vi "写入差值数据excel.vi"(7 "IN":i32=129, 8 "error in (no error)":errorcluster, 9 "COM":i32=4, 10 "差值限":dbl, 11 "NI_report in":refnum<class "NI_report.lvclass">) -> (0 "error out":errorcluster, 3 "NI_report out":refnum<class "NI_report.lvclass">)   [LabVIEW 2015]
uses:
  <vilib>/Utility/NIReport.llb/NI_report.lvclass
  <vilib>/addons/_office/excel.llb/Excel Easy Table (str).vi
  <vilib>/Utility/NIReport.llb/Excel/NI_Excel.lvclass
  <vilib>/addons/_office/NI_ReportGenerationToolkit.lvlib
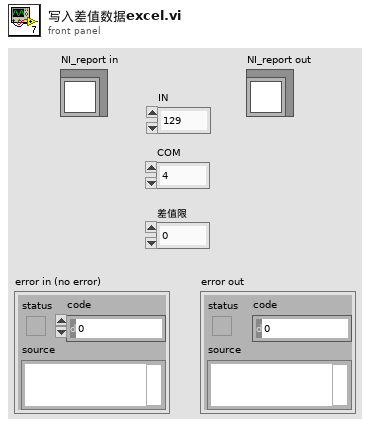
[diagram p1: front panel]
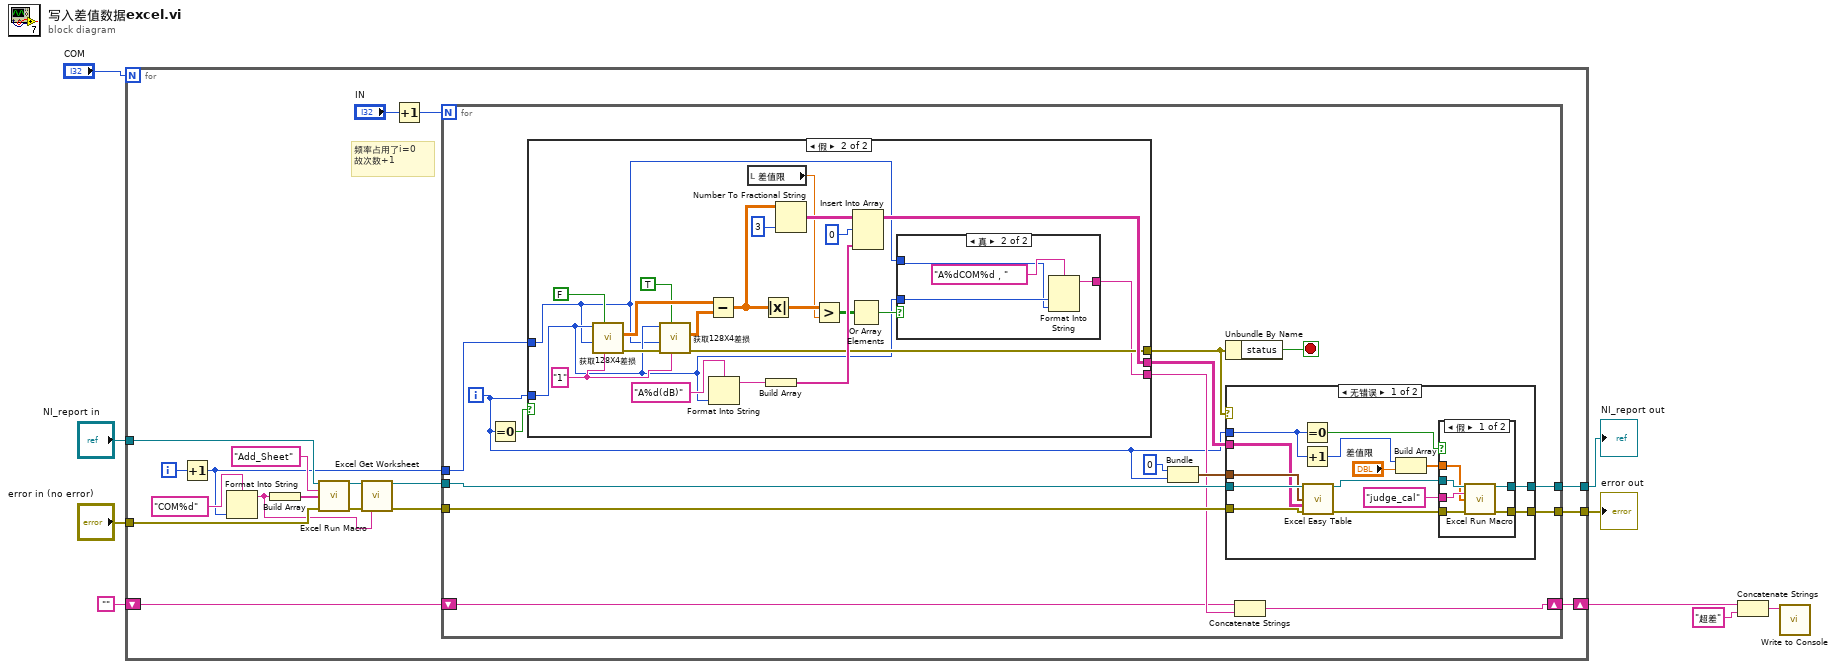
[diagram p0: block diagram]
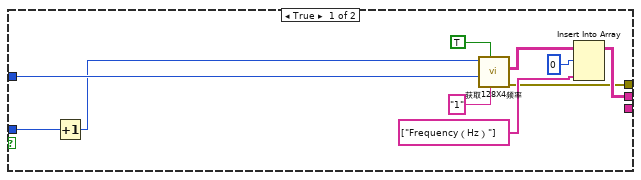
[diagram p2: hidden frame]
diagram:
  n1 = for {
    N: "COM" -> [_]
    tunnel: "NI_report in" -> [w25]
    tunnel: "error in (no error)" -> [w24]
    tunnel: [w14] -> w8
    tunnel: [w13] -> w9
    shift-right: [w12] -> w3
    shift-left: "" -> [w11]
    i -> [w20]
    # "频率占用了i=0\n故次数+1"
    n2 = Increment(x=w20) -> (x+1=w17:i32)
    n3 = Format Into String(format string="COM%d" ("style"), w17) -> (resulting string=w18:string)  [unwired: 2 in, 1 out]
    n4 = Build Array(w18) -> (w22:string[])
    n5 = call <vilib>:"Excel Run Macro.vi"("report in"=w25, "macro name"="Add_Sheet", "parameters"=w22, "error in (no error)"=w24) -> ("report out"=w27:refnum<class "NI_report.lvclass">, "error out"=w23:errorcluster)  [unwired: 9 in, 1 out]
    n6 = call <vilib>:"Excel Get Worksheet.vi"("report in"=w27, "error in (no error)"=w23, "name (\"\")"=w18) -> ("report out"=w16:refnum<class "NI_report.lvclass">, "error out"=w15:errorcluster)  [unwired: 11 in]
    n7 = Increment(x="IN") -> (x+1=w10:i32)
    n8 = for {
      N: w10 -> [_]
      tunnel: w17 -> [w34]
      tunnel: w16 -> [w42]
      tunnel: w15 -> [w41]
      tunnel: [w37] -> w14
      tunnel: [w36] -> w13
      shift-right: [w30] -> w12
      shift-left: w11 -> [w29]
      i -> [w28]
      stop <- w33 stop-if-true
      n9 = Equal To 0?(x=w28) -> (x = 0?=w35:bool)
      n10 = case shown="假" w35 {
        tunnel: w28 -> [w44 w56]
        tunnel: [w51 w63] -> w40
        tunnel: w34 -> [w49 w55]
        tunnel: [w45 w62] -> w32
        tunnel: [_ w54] -> w31
        frame True {
          n11 = Increment(x=w44) -> (x+1=w43:i32)
          n12 = call "获取128X4频率.vi"("testType"="1", "ref"=TRUE, "COM"=w49, "A"=w43) -> ("error out"=w45:errorcluster, "Freq&S21"=w46:string[][])  [unwired: 6 in]
          n13 = Insert Into Array(array=w46, index (row)=0, new element=string[] ["Frequency（Hz）"] ("new element/subarray")) -> (w51:string[][])  [unwired: 1 in]
        }
        frame False {
          w70 = "1" ("testType")
          n14 = call "获取128X4差损.vi"("testType"=w70, "ref"=FALSE, "COM"=w55, "A"=w56) -> ("error out"=w68:errorcluster, "S21"=w67:dbl[][])  [unwired: 6 in]
          n15 = call "获取128X4差损.vi"("testType"=w70, "ref"=TRUE, "error in (no error)"=w68, "COM"=w55, "A"=w56) -> ("error out"=w62:errorcluster, "S21"=w66:dbl[][])  [unwired: 5 in]
          n16 = Subtract(x=w67, y=w66) -> (x-y=w61:dbl[][])
          n17 = Format Into String(format string="A%d(dB)", w56) -> (resulting string=w72:string)  [unwired: 2 in, 1 out]
          n18 = local read "差值限"() -> (w59:dbl)
          n19 = Absolute Value(x=w61) -> (abs(x)=w60:dbl[][])
          n20 = Build Array(w72) -> (w71:string[])
          n21 = Number To Fractional String(number=w61, precision (6)=i16 3) -> (F-format string=w64:string[][])  [unwired: 2 in]
          n22 = Greater?(x=w60, y=w59) -> (0:w58:bool[][])
          n23 = Or Array Elements(Boolean array=w58) -> (logical OR=w57:bool)
          n24 = Insert Into Array(array=w64, index (row)=0, new element=w71) -> (w63:string[][])  [unwired: 1 in]
          n25 = case shown="真" w57 {
            tunnel: w56 -> [_ w77]
            tunnel: w55 -> [_ w76]
            tunnel: [_ w75] -> w54
            frame False {
            }
            frame True {
              n26 = Format Into String(format string="A%dCOM%d，", w77, w76) -> (resulting string=w75:string)  [unwired: 2 in, 1 out]
            }
          }
        }
      }
      n27 = Bundle(0, w28) -> (w38:cluster{i32, i32})  [unwired: 1 in]
      n28 = Unbundle By Name(w32) -> ("status"=w33:bool)
      n29 = case shown="无错误" w32 {
        tunnel: w42 -> [w92 w102]
        tunnel: w41 -> [w91 w101]
        tunnel: w40 -> [w89 _]
        tunnel: w38 -> [w90 _]
        tunnel: [w87 w102] -> w37
        tunnel: [w86 w101] -> w36
        tunnel: w28 -> [w80 _]
        frame No Error {
          n30 = Equal To 0?(x=w80) -> (x = 0?=w79:bool)
          n31 = Increment(x=w80) -> (x+1=w82:i32)
          n32 = call-poly <vilib>:"Excel Easy Table.vi"("report in"=w92, "start (0, 0)"=w90, "text data"=w89, "error in (no error)"=w91) -> ("report out"=w88:refnum<class "NI_report.lvclass">, "error out"=w85:errorcluster)  [unwired: 7 in, 3 out]
          n33 = Build Array(w82, "差值限") -> (w81:dbl[])
          n34 = case shown="假" w79 {
            tunnel: w88 -> [w98 w100]
            tunnel: [w97 w100] -> w87
            tunnel: [w96 w99] -> w86
            tunnel: w85 -> [w95 w99]
            tunnel: "judge_cal" ("macro name") -> [w94 _]
            tunnel: w81 -> [w93 _]
            frame False {
              n35 = call <vilib>:"Excel Run Macro.vi"("report in"=w98, "macro name"=w94, "parameters"=w93, "error in (no error)"=w95) -> ("report out"=w97:refnum<class "NI_report.lvclass">, "error out"=w96:errorcluster)  [unwired: 9 in, 1 out]
            }
            frame True {
            }
          }
        }
        frame Error {
        }
      }
      n36 = Concatenate Strings(w29, w31) -> (w30:string)
    }
  }
  "error out" <- w9
  "NI_report out" <- w8
  n37 = Concatenate Strings(w3, "超差" ("string")) -> (w2:string)
  n38 = call "Write to Console.vi"("Input"=w2) -> ()  [unwired: 10 in, 1 out]
